vi "Get Controller .NET.vi"(11 "Custom Events in":refnum<class "Custom Events.lvclass">) -> (2 "CustomEvents .NET":refnum<k24>, 3 "Custom Events out":refnum<class "Custom Events.lvclass">)   [LabVIEW 2024, in "SourceGrid.lvlib" / "Custom Events.lvclass"]
uses:
  Custom Events.lvclass
  D:/git/Sourcegrid-LabVIEW/dll/SourceGrid.dll
  dll/SourceGrid.dll
  Custom Events.lvclass/Custom Events.ctl
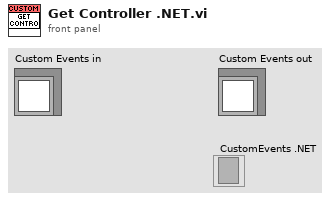
[diagram p1: front panel]
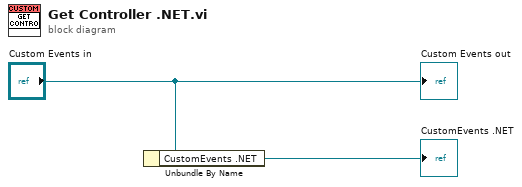
[diagram p0: block diagram]
diagram:
  n1 = Unbundle By Name("Custom Events in") -> ("CustomEvents .NET"=→"CustomEvents .NET":refnum<k24>)
  "Custom Events out" <- "Custom Events in"
